vi "CheckNTData.vi"(10 "ValToCheck":dbl, 11 "Mode":enum16{"Start Loop", "End Loop"}(ring)) -> ()   [LabVIEW 2018]
uses:
  <vilib>/Rock Robotics/Network Tables/NT Write Boolean.vi
  Swerve/SwerveGlobals.vi
  <vilib>/Rock Robotics/Network Tables/NT Read Boolean.vi
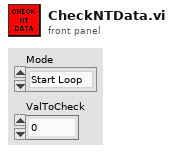
[diagram p1: front panel]
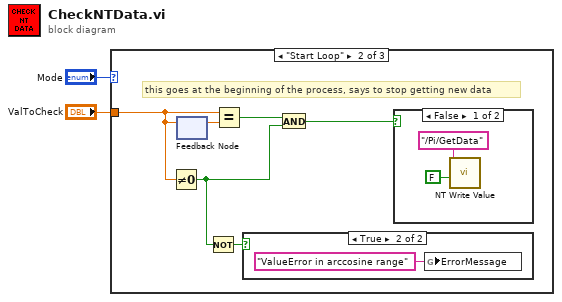
[diagram p0: block diagram]
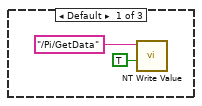
[diagram p2: hidden frame]
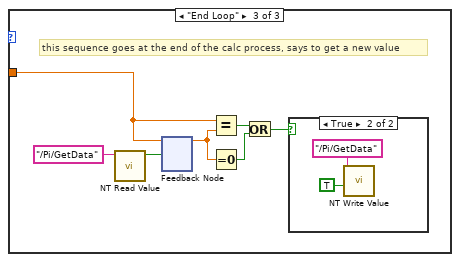
[diagram p5: hidden frame]
diagram:
  n1 = case shown="\"Start Loop\"" "Mode" {
    tunnel: "ValToCheck" -> [_ w8 w14]
    frame Default {
      n2 = call-poly <vilib>:"NT Write Value.vi"("Boolean"=TRUE, "Name"="/Pi/GetData" ("Client Name")) -> ()  [unwired: 9 in, 1 out]
    }
    frame "Start Loop" {
      # "this goes at the beginning of the process, says to stop getting new data"
      n3 = Not Equal To 0?(x=w8) -> (x != 0?=w5:bool)
      n4 = feedback #1() -> (w10:dbl)  [unwired: 1 in]
      n5 = feedback-in #1(w8) -> ()
      n6 = Not(x=w5) -> (.not. x?=w6:bool)
      n7 = Equal?(x=w8, y=w10) -> (x = y?=w9:bool)
      n8 = case shown="True" w6 {
        frame False {
        }
        frame True {
          n9 = global write "SwerveGlobals.vi" "ErrorMessage"("ValueError in arccosine range" ("ErrorMessage")) -> ()
        }
      }
      n10 = And(x=w9, y=w5) -> (x .and. y?=w7:bool)
      n11 = case shown="False" w7 {
        frame False {
          n12 = call-poly <vilib>:"NT Write Value.vi"("Boolean"=FALSE, "Name"="/Pi/GetData" ("Client Name")) -> ()  [unwired: 9 in, 1 out]
        }
        frame True {
        }
      }
    }
    frame "End Loop" {
      # "this sequence goes at the end of the calc process, says to get a new value"
      n13 = call-poly <vilib>:"NT Read Value.vi"("Name"="/Pi/GetData" ("Client Name")) -> ("Boolean"=w15:bool)  [unwired: 9 in, 1 out]
      n14 = feedback #2() -> (w20:dbl)  [unwired: 1 in]
      n15 = feedback-in #2(w14, w15) -> ()
      n16 = Equal?(x=w14, y=w20) -> (x = y?=w19:bool)
      n17 = Equal To 0?(x=w20) -> (x = 0?=w18:bool)
      n18 = Or(x=w19, y=w18) -> (x .or. y?=w17:bool)
      n19 = case shown="True" w17 {
        frame False {
        }
        frame True {
          n20 = call-poly <vilib>:"NT Write Value.vi"("Boolean"=TRUE, "Name"="/Pi/GetData" ("Client Name")) -> ()  [unwired: 9 in, 1 out]
        }
      }
    }
  }
